vi "Config Process.vi"(8 "error in (no error)":errorcluster, 11 "View Model":T1) -> (0 "error out":errorcluster, 3 "View Model":T1)   [LabVIEW 2017]
doc: "Provides all functions for operates with data records."
uses:
  View Model/Controls/View Model.ctl
  Controls/Config Model.ctl
  Controls/Config Commands.ctl
  Controls/Congif Data.ctl
  View Model/Controls/Shared Model.ctl
  Error Handler/Controls/Error Model.ctl
  Error Handler/Controls/Error Data.ctl
  Error Handler/Controls/Error Type.ctl
  Car Wash Controller/Controls/Car Wash Model.ctl
  Car Wash Controller/Controls/Controller Overhead.ctl
  Car Wash Controller/Controls/Vehicle Location.ctl
  Car Wash Controller/Controls/Car Wash States.ctl
  Car Wash Controller/Controls/CarWash CMD.ctl
  Views/Wash Display Console View/Controls/Car Wash Indicators.ctl
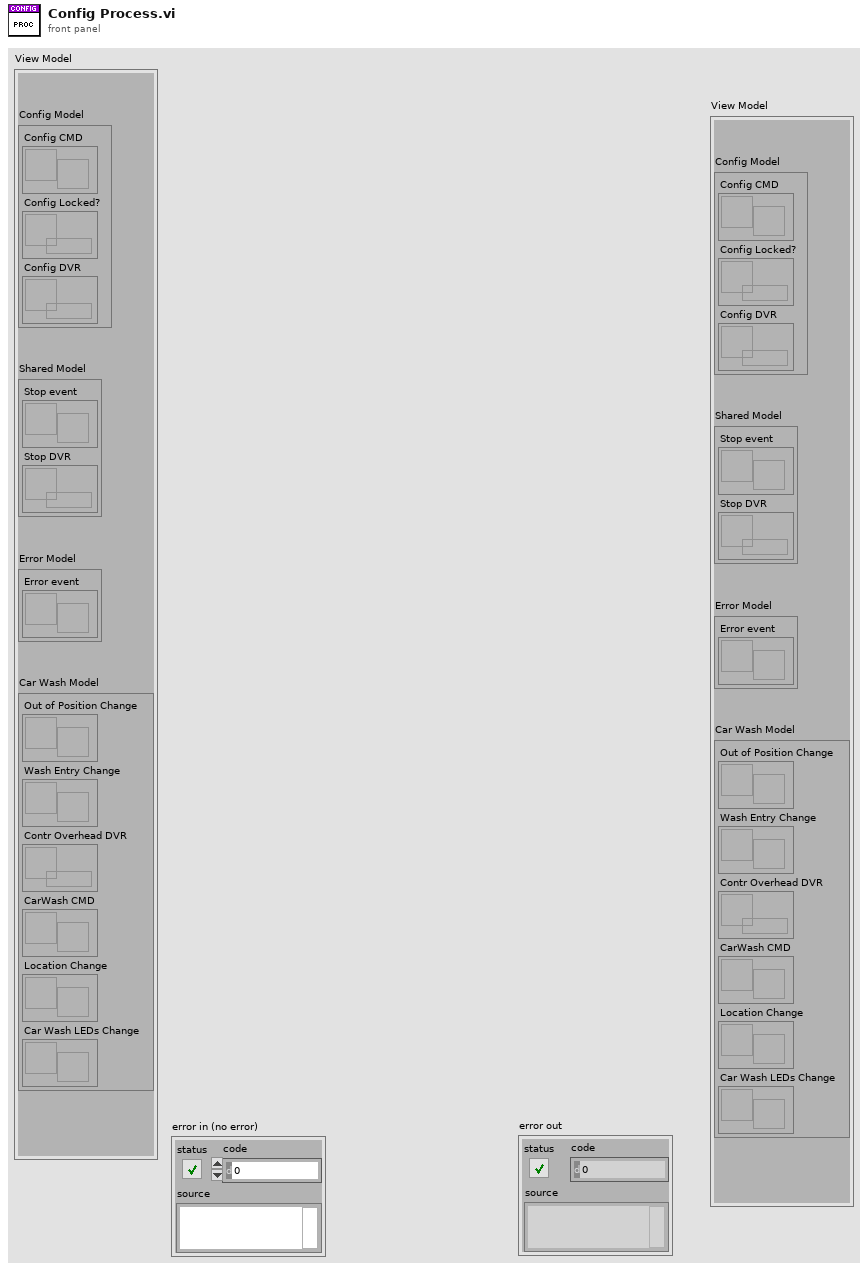
[diagram p1: front panel]
types:
  T1 = typedef "View Model.ctl" = cluster{"Config Model":T2, "Shared Model":T3, "Error Model":T4, "Car Wash Model":T5}
  T2 = typedef "Config Model.ctl" = cluster{"Config CMD":refnum<user-event>, "Config Locked?":refnum<data-value>, "Config DVR":refnum<data-value>}
  T3 = typedef "Shared Model.ctl" = cluster{"Stop event":refnum<user-event>, "Stop DVR":refnum<data-value>}
  T4 = typedef "Error Model.ctl" = cluster{"Error event":refnum<user-event>}
  T5 = typedef "Car Wash Model.ctl" = cluster{"Out of Position Change":refnum<user-event>, "Wash Entry Change":refnum<user-event>, "Contr Overhead DVR":refnum<data-value>, "CarWash CMD":refnum<user-event>, "Location Change":refnum<user-event>, "Car Wash LEDs Change":refnum<user-event>}
  T6 = typedef "Congif Data.ctl" = cluster{"Wash Step":string, "Station":string, "Step Duration":u32}
  T7 = typedef "Config Commands.ctl" = enum16{"Read records", "Query timing data", "Insert new data records", "Update data records"}
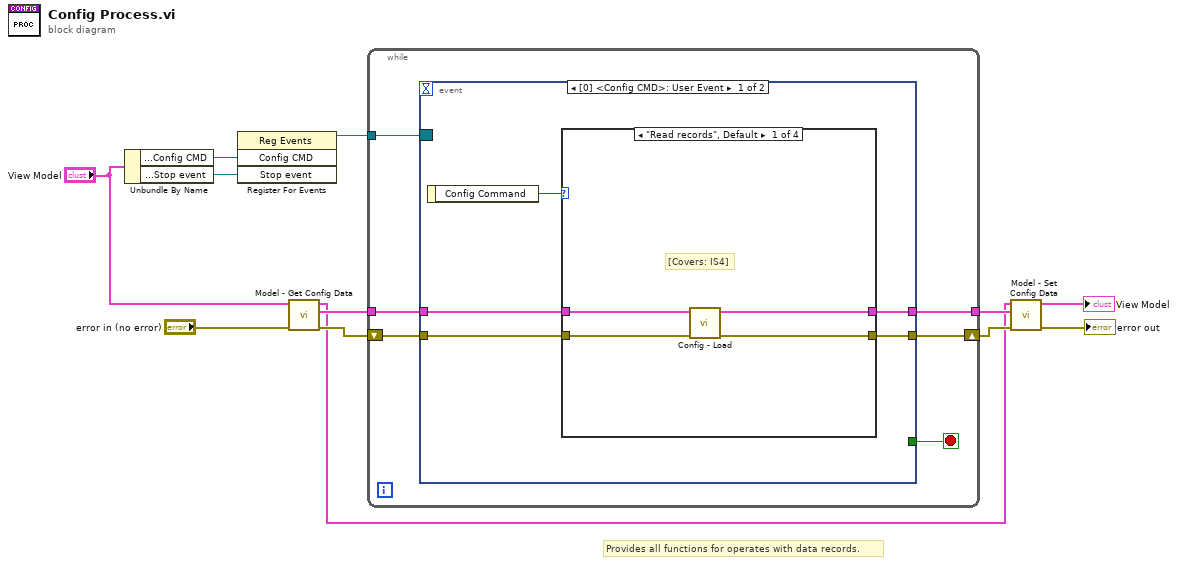
[diagram p0: block diagram]
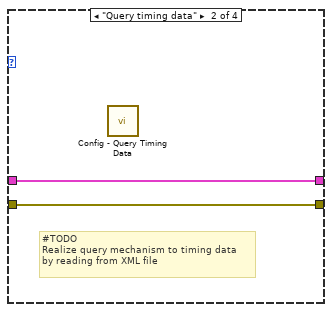
[diagram p2: hidden frame]
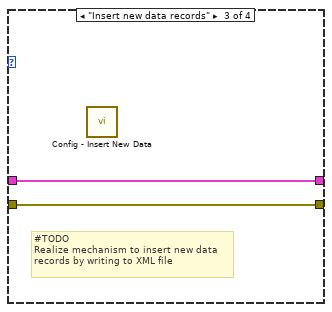
[diagram p3: hidden frame]
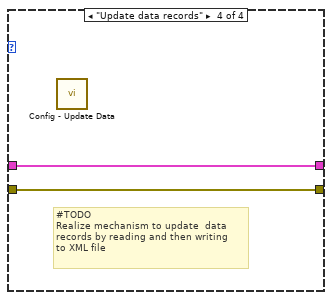
[diagram p4: hidden frame]
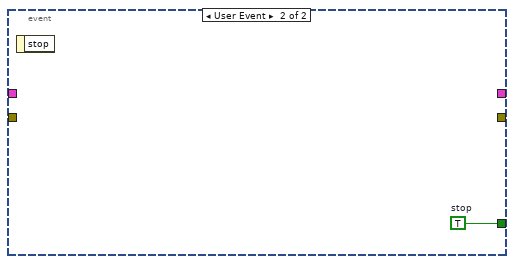
[diagram p5: hidden frame]
diagram:
  # "Provides all functions for operates with data records."
  n1 = Unbundle By Name("View Model") -> ("Config Model.Config CMD"=w12:refnum<user-event>, "Shared Model.Stop event"=w10:refnum<user-event>)
  n2 = register-events(w12, w10) -> (reference out=w11:refnum<event-registration>)  [unwired: 2 in, 1 out]
  n3 = call "Model - Get Config Data.vi"("error in (no error)"="error in (no error)", "View Model"="View Model") -> ("error out"=w7:errorcluster, "Config Data"=w6:T6[], "View Model"=w2:T1)  [unwired: 7 in]
  n4 = while {
    tunnel: w11 -> [w18]
    shift-right: [w15] -> w4
    shift-left: w7 -> [w17]
    tunnel: w6 -> [w16]
    tunnel: [w14] -> w5
    stop <- w13 stop-if-true
    n5 = event shown="[0] <Config CMD>: User Event" {
      selector: w18 -> [_ _]
      dyn-events: _ -> [_ _]
      timeout: _ -> [_ _]
      tunnel: w17 -> [w22 _]
      tunnel: w16 -> [w21 _]
      tunnel: [w20 _] -> w15
      tunnel: [w19 _] -> w14
      tunnel: [_ w34] -> w13
      event User Event {
        n6 = event-data() -> ("Config Command"=w23:T7)  [unwired: 1 in]
        n7 = case shown="\"Read records\", Default" w23 {
          tunnel: w22 -> [w27 w29 w31 w33]
          tunnel: w21 -> [w24 w28 w30 w32]
          tunnel: [w26 w29 w31 w33] -> w20
          tunnel: [w25 w28 w30 w32] -> w19
          frame "Read records", Default {
            # "[Covers: IS4]"
            n8 = call "Config - Load.vi"("error in (no error)"=w27, "Config Data"=w24) -> ("error out"=w26:errorcluster, "Config Data"=w25:T6[])  [unwired: 8 in]
          }
          frame "Query timing data" {
            # "#TODO\nRealize query mechanism to timing data\nby reading from XML file"
            n9 = call "Config - Query Timing Data.vi"() -> ()  [unwired: 10 in, 2 out]
          }
          frame "Insert new data records" {
            # "#TODO\nRealize mechanism to insert new data\nrecords by writing to XML file"
            n10 = call "Config - Insert New Data.vi"() -> ()  [unwired: 10 in, 2 out]
          }
          frame "Update data records" {
            # "#TODO\nRealize mechanism to update  data\nrecords by reading and then writing \nto XML file"
            n11 = call "Config - Update Data.vi"() -> ()  [unwired: 10 in, 2 out]
          }
        }
      }
      event User Event {
        w34 = TRUE  # stop
        n12 = event-data() -> ()  [unwired: 1 in, 1 out]
      }
    }
  }
  n13 = call "Model - Set Config Data.vi"("error in (no error)"=w4, "Config Data"=w5, "View Model"=w2) -> ("error out"=→"error out":errorcluster, "View Model"=→"View Model":T1)  [unwired: 7 in]
